vi "GLOBAL.vi"() -> ()   [LabVIEW 2018]
panel:
  in  "BREAK":bool
  in  "STOP":bool
  in  "quit":bool
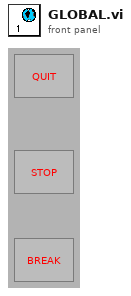
[diagram p1: front panel]
diagram:
